vi "bangBangNavigation.vi"(0 "Game":refnum<class "Game.lvclass">, 1 "RobotRef":refnum<class "Robot.lvclass">[](array[class]), 5 "error in (no error)":errorcluster) -> (16 "RoboRef":refnum<class "Robot.lvclass">[](array[class]), 17 "NaN?":bool, 18 "NewNaN?":bool, 19 "error out":errorcluster)   [LabVIEW 2020, in "Game.lvclass"]
uses:
  Game.lvclass
  Robot_class/Robot.lvclass
  Navigation/Controls/typeOfUse.ctl
  Robot_class/Robot.lvclass/Robot.ctl
  Robot_class/Write v_ang.vi
  Robot_class/Write v_norm.vi
  Robot_class/Write v_tang.vi
  Robot_class/Read id.vi
  Robot_class/Read v_tang.vi
  Robot_class/Read v_norm.vi
  Robot_class/Read v_ang.vi
panel:
  in  "delta":dbl=0.2
  in  "desired_vtang":dbl=1.0
  in  "est_vtang":dbl=2.0
  out "array":dbl[][](array[numeric])
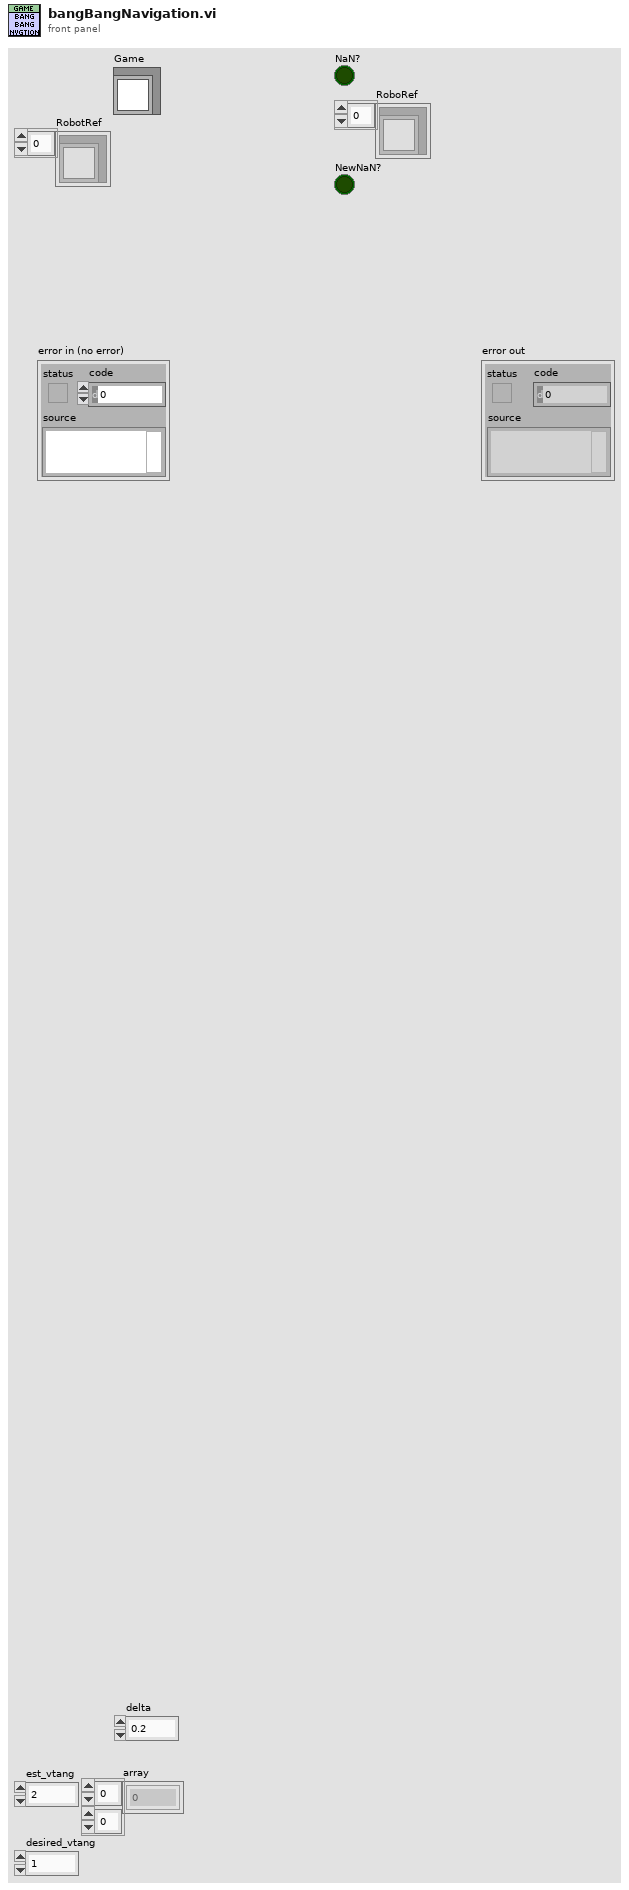
[diagram p1: front panel]
types:
  T1 = typedef "typeOfUse.ctl" = enum16{"Navigation", "grSimTest"}
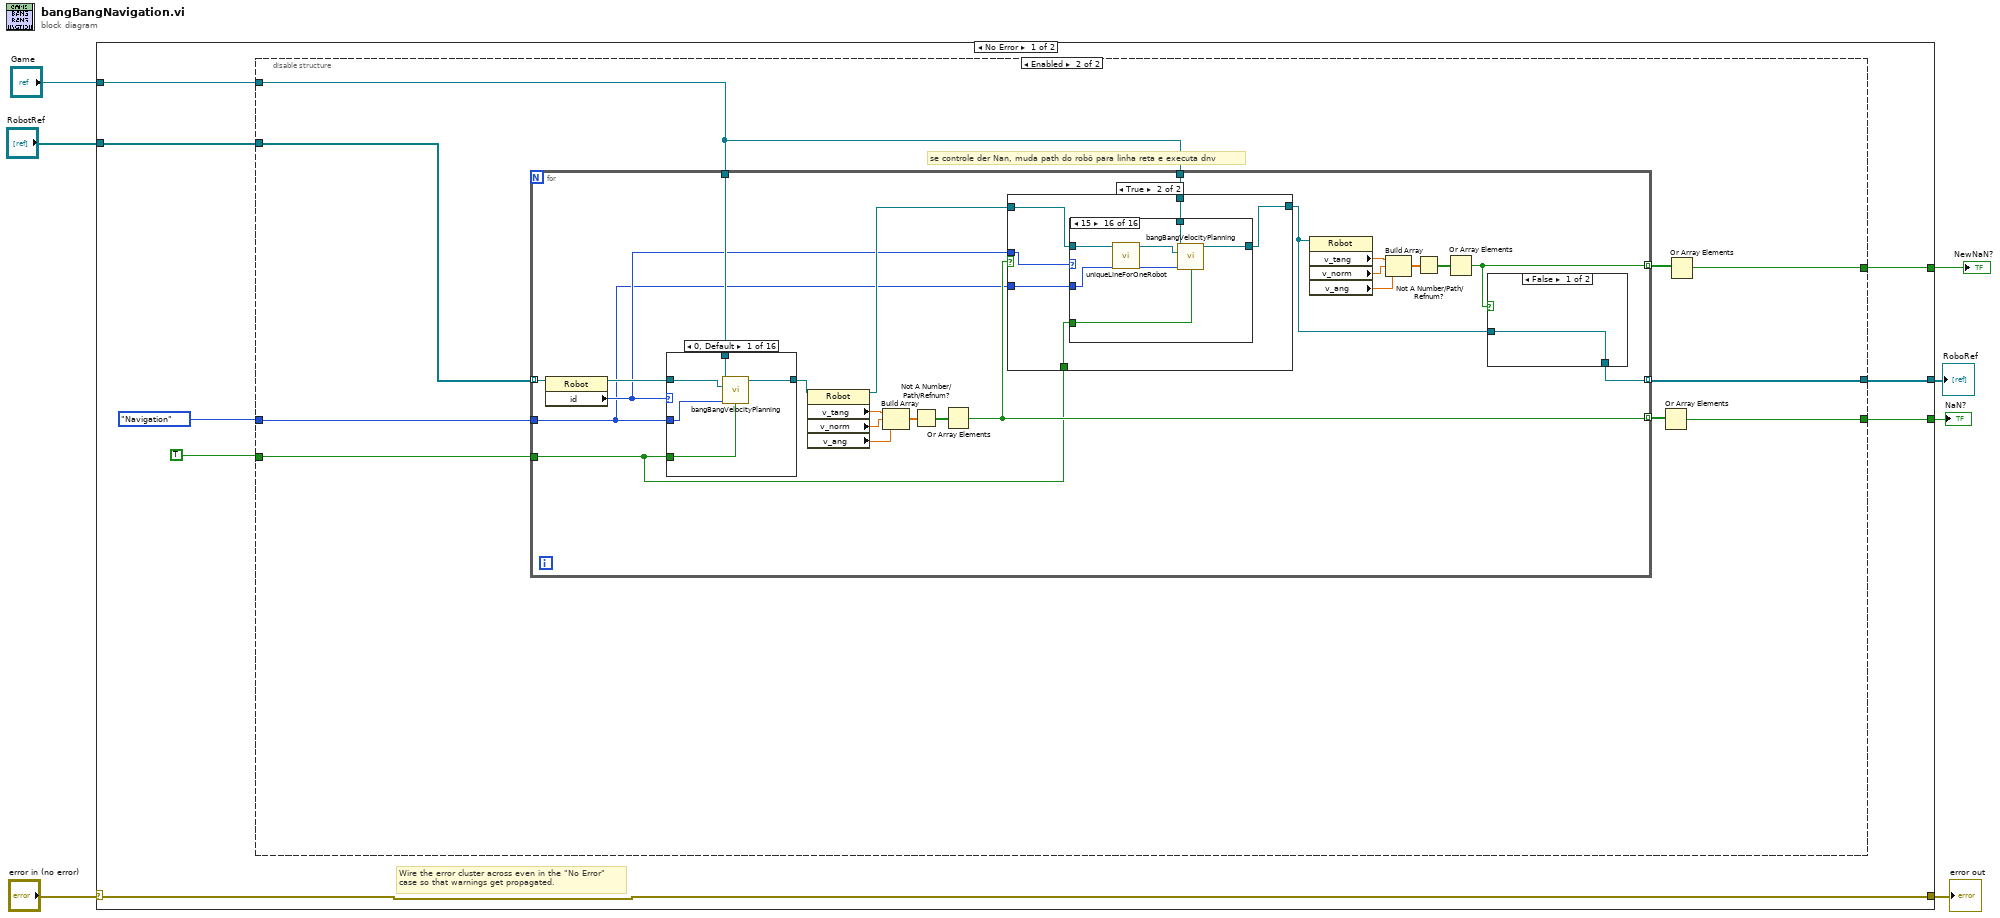
[diagram p0: block diagram]
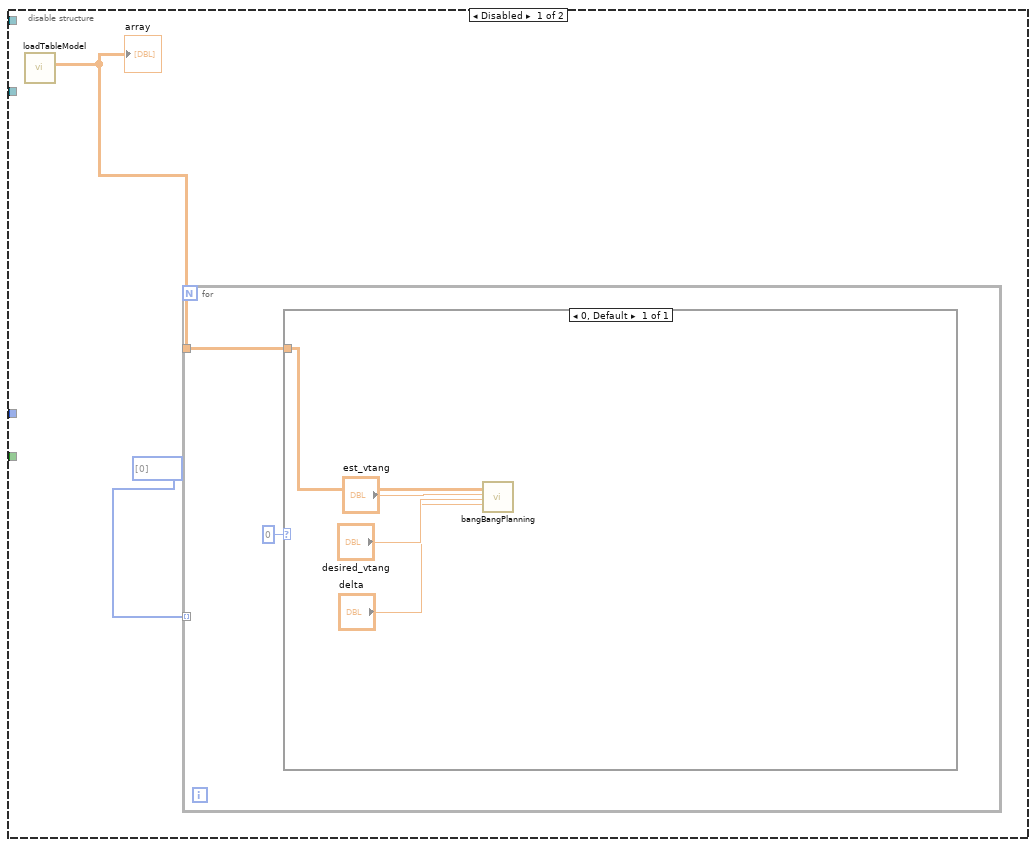
[diagram p2: hidden frame]
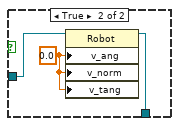
[diagram p3: hidden frame]
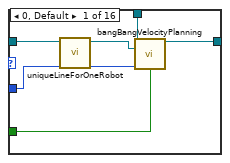
[diagram p5: hidden frame]
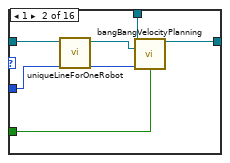
[diagram p6: hidden frame]
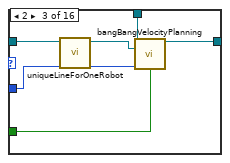
[diagram p7: hidden frame]
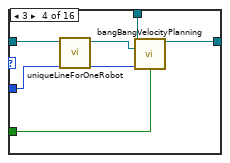
[diagram p8: hidden frame]
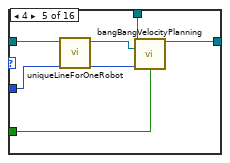
[diagram p9: hidden frame]
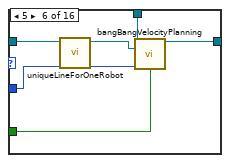
[diagram p10: hidden frame]
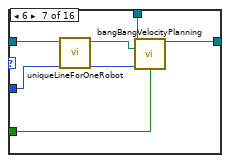
[diagram p11: hidden frame]
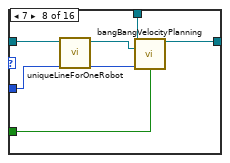
[diagram p12: hidden frame]
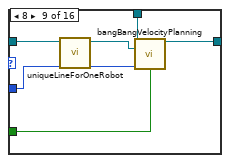
[diagram p13: hidden frame]
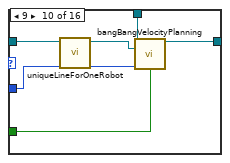
[diagram p14: hidden frame]
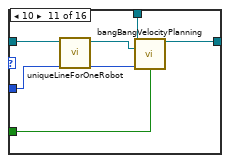
[diagram p15: hidden frame]
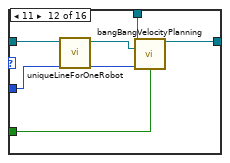
[diagram p16: hidden frame]
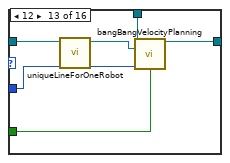
[diagram p17: hidden frame]
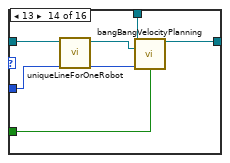
[diagram p18: hidden frame]
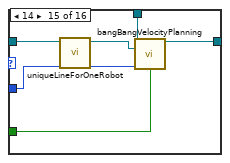
[diagram p19: hidden frame]
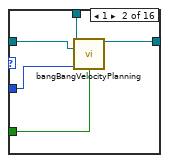
[diagram p20: hidden frame]
diagram:
  n1 = case shown="No Error" "error in (no error)" {
    selector: "error in (no error)" -> [w15 w243]
    tunnel: [w15 w243] -> w6
    tunnel: [w12 _] -> w5
    tunnel: [w11 _] -> w4
    tunnel: "RobotRef" -> [w10 _]
    tunnel: "Game" -> [w9 _]
    tunnel: [w8 _] -> w1
    frame No Error {
      # "Wire the error cluster across even in the \"No Error\"\ncase so that warnings get propagated."
      n2 = disable-structure shown="Enabled" {
        disable-tunnel: TRUE ("start") -> [_ w32]
        disable-tunnel: typeOfUse."Navigation" ("type_of_use") -> [_ w31]
        disable-tunnel: [_ w29] -> w12
        disable-tunnel: [_ w28] -> w11
        disable-tunnel: w10 -> [_ w27]
        disable-tunnel: w9 -> [_ w26]
        disable-tunnel: [_ w24] -> w8
        frame Disabled {
          n3 = call "loadTableModel.vi"() -> ("array"=w17:dbl[][])  [unwired: 9 in, 2 out]
          "array" <- w17
          n4 = for {
            tunnel: w17 -> [w19]
            tunnel: i32[] [0] -> [_] mode=indexing
            n5 = case shown="0, Default" u32 0 ("id") {
              tunnel: w19 -> [w23]
              frame 0, Default {
                n6 = call "bangBangPlanning.vi"("array"=w23, "est_vtang"="est_vtang", "desired_vtang"="desired_vtang", "delta"="delta") -> ()  [unwired: 14 in, 2 out]
              }
            }
          }
        }
        frame Enabled {
          # "se controle der Nan, muda path do robô para linha reta e executa dnv"
          n7 = for {
            tunnel: w27 -> [w55] mode=indexing
            tunnel: w32 -> [w41]
            tunnel: [w33] -> w28 mode=indexing
            tunnel: w31 -> [w42]
            tunnel: [w47] -> w30 mode=indexing
            tunnel: w26 -> [w45]
            tunnel: w26 -> [w43]
            tunnel: [w35] -> w25 mode=indexing
            n8 = property class="Robot"(reference=w55) -> (reference out=w54:refnum<class "Robot.lvclass">, "id"=w44:i32)  [unwired: 1 in, 1 out]
            n9 = case shown="0, Default" w44 {
              tunnel: w54 -> [w164 w169 w174 w179 w184 w189 w194 w199 w204 w209 w214 w219 w224 w229 w234 w239]
              tunnel: w41 -> [w167 w172 w177 w182 w187 w192 w197 w202 w207 w212 w217 w222 w227 w232 w237 w242]
              tunnel: [w166 w171 w176 w181 w186 w191 w196 w201 w206 w211 w216 w221 w226 w231 w236 w241] -> w53
              tunnel: w42 -> [w165 w170 w175 w180 w185 w190 w195 w200 w205 w210 w215 w220 w225 w230 w235 w240]
              tunnel: w45 -> [w163 w168 w173 w178 w183 w188 w193 w198 w203 w208 w213 w218 w223 w228 w233 w238]
              frame 0, Default {
                n10 = call "bangBangVelocityPlanning.vi"("Game"=w163, "Robot in"=w164, "type_of_use"=w165, "start"=w167) -> ("Robot out"=w166:refnum<class "Robot.lvclass">)  [unwired: 9 in, 2 out]
              }
              frame 1 {
                n11 = call "bangBangVelocityPlanning.vi"("Game"=w168, "Robot in"=w169, "type_of_use"=w170, "start"=w172) -> ("Robot out"=w171:refnum<class "Robot.lvclass">)  [unwired: 9 in, 2 out]
              }
              frame 2 {
                n12 = call "bangBangVelocityPlanning.vi"("Game"=w173, "Robot in"=w174, "type_of_use"=w175, "start"=w177) -> ("Robot out"=w176:refnum<class "Robot.lvclass">)  [unwired: 9 in, 2 out]
              }
              frame 3 {
                n13 = call "bangBangVelocityPlanning.vi"("Game"=w178, "Robot in"=w179, "type_of_use"=w180, "start"=w182) -> ("Robot out"=w181:refnum<class "Robot.lvclass">)  [unwired: 9 in, 2 out]
              }
              frame 4 {
                n14 = call "bangBangVelocityPlanning.vi"("Game"=w183, "Robot in"=w184, "type_of_use"=w185, "start"=w187) -> ("Robot out"=w186:refnum<class "Robot.lvclass">)  [unwired: 9 in, 2 out]
              }
              frame 5 {
                n15 = call "bangBangVelocityPlanning.vi"("Game"=w188, "Robot in"=w189, "type_of_use"=w190, "start"=w192) -> ("Robot out"=w191:refnum<class "Robot.lvclass">)  [unwired: 9 in, 2 out]
              }
              frame 6 {
                n16 = call "bangBangVelocityPlanning.vi"("Game"=w193, "Robot in"=w194, "type_of_use"=w195, "start"=w197) -> ("Robot out"=w196:refnum<class "Robot.lvclass">)  [unwired: 9 in, 2 out]
              }
              frame 7 {
                n17 = call "bangBangVelocityPlanning.vi"("Game"=w198, "Robot in"=w199, "type_of_use"=w200, "start"=w202) -> ("Robot out"=w201:refnum<class "Robot.lvclass">)  [unwired: 9 in, 2 out]
              }
              frame 8 {
                n18 = call "bangBangVelocityPlanning.vi"("Game"=w203, "Robot in"=w204, "type_of_use"=w205, "start"=w207) -> ("Robot out"=w206:refnum<class "Robot.lvclass">)  [unwired: 9 in, 2 out]
              }
              frame 9 {
                n19 = call "bangBangVelocityPlanning.vi"("Game"=w208, "Robot in"=w209, "type_of_use"=w210, "start"=w212) -> ("Robot out"=w211:refnum<class "Robot.lvclass">)  [unwired: 9 in, 2 out]
              }
              frame 10 {
                n20 = call "bangBangVelocityPlanning.vi"("Game"=w213, "Robot in"=w214, "type_of_use"=w215, "start"=w217) -> ("Robot out"=w216:refnum<class "Robot.lvclass">)  [unwired: 9 in, 2 out]
              }
              frame 11 {
                n21 = call "bangBangVelocityPlanning.vi"("Game"=w218, "Robot in"=w219, "type_of_use"=w220, "start"=w222) -> ("Robot out"=w221:refnum<class "Robot.lvclass">)  [unwired: 9 in, 2 out]
              }
              frame 12 {
                n22 = call "bangBangVelocityPlanning.vi"("Game"=w223, "Robot in"=w224, "type_of_use"=w225, "start"=w227) -> ("Robot out"=w226:refnum<class "Robot.lvclass">)  [unwired: 9 in, 2 out]
              }
              frame 13 {
                n23 = call "bangBangVelocityPlanning.vi"("Game"=w228, "Robot in"=w229, "type_of_use"=w230, "start"=w232) -> ("Robot out"=w231:refnum<class "Robot.lvclass">)  [unwired: 9 in, 2 out]
              }
              frame 14 {
                n24 = call "bangBangVelocityPlanning.vi"("Game"=w233, "Robot in"=w234, "type_of_use"=w235, "start"=w237) -> ("Robot out"=w236:refnum<class "Robot.lvclass">)  [unwired: 9 in, 2 out]
              }
              frame 15 {
                n25 = call "bangBangVelocityPlanning.vi"("Game"=w238, "Robot in"=w239, "type_of_use"=w240, "start"=w242) -> ("Robot out"=w241:refnum<class "Robot.lvclass">)  [unwired: 9 in, 2 out]
              }
            }
            n26 = property class="Robot"(reference=w53) -> (reference out=w46:refnum<class "Robot.lvclass">, "v_tang"=w52:dbl, "v_norm"=w51:dbl, "v_ang"=w49:dbl)  [unwired: 1 in, 1 out]
            n27 = Build Array(w52, w51, w49) -> (w50:dbl[])
            n28 = Not A Number/Path/Refnum?(number/path/refnum=w50) -> (NaN/Path/Refnum?=w48:bool[])
            n29 = Or Array Elements(Boolean array=w48) -> (logical OR=w47:bool)
            n30 = case shown="True" w47 {
              tunnel: w46 -> [w60 w65]
              tunnel: [w60 w61] -> w34
              tunnel: w44 -> [_ w66]
              tunnel: w43 -> [_ w64]
              tunnel: w42 -> [_ w63]
              tunnel: w41 -> [_ w62]
              frame False {
              }
              frame True {
                n31 = case shown="15" w66 {
                  tunnel: w65 -> [w68 w74 w80 w86 w92 w98 w104 w110 w116 w122 w128 w134 w140 w146 w152 w158]
                  tunnel: w62 -> [w72 w78 w84 w90 w96 w102 w108 w114 w120 w126 w132 w138 w144 w150 w156 w162]
                  tunnel: [w71 w77 w83 w89 w95 w101 w107 w113 w119 w125 w131 w137 w143 w149 w155 w161] -> w61
                  tunnel: w63 -> [w70 w76 w82 w88 w94 w100 w106 w112 w118 w124 w130 w136 w142 w148 w154 w160]
                  tunnel: w64 -> [w69 w75 w81 w87 w93 w99 w105 w111 w117 w123 w129 w135 w141 w147 w153 w159]
                  frame 0, Default {
                    n32 = call "uniqueLineForOneRobot.vi"("Robot in"=w68) -> ("Robot out"=w67:refnum<class "Robot.lvclass">)  [unwired: 10 in]
                    n33 = call "bangBangVelocityPlanning.vi"("Game"=w69, "Robot in"=w67, "type_of_use"=w70, "start"=w72) -> ("Robot out"=w71:refnum<class "Robot.lvclass">)  [unwired: 9 in, 2 out]
                  }
                  frame 1 {
                    n34 = call "uniqueLineForOneRobot.vi"("Robot in"=w74) -> ("Robot out"=w73:refnum<class "Robot.lvclass">)  [unwired: 10 in]
                    n35 = call "bangBangVelocityPlanning.vi"("Game"=w75, "Robot in"=w73, "type_of_use"=w76, "start"=w78) -> ("Robot out"=w77:refnum<class "Robot.lvclass">)  [unwired: 9 in, 2 out]
                  }
                  frame 2 {
                    n36 = call "uniqueLineForOneRobot.vi"("Robot in"=w80) -> ("Robot out"=w79:refnum<class "Robot.lvclass">)  [unwired: 10 in]
                    n37 = call "bangBangVelocityPlanning.vi"("Game"=w81, "Robot in"=w79, "type_of_use"=w82, "start"=w84) -> ("Robot out"=w83:refnum<class "Robot.lvclass">)  [unwired: 9 in, 2 out]
                  }
                  frame 3 {
                    n38 = call "uniqueLineForOneRobot.vi"("Robot in"=w86) -> ("Robot out"=w85:refnum<class "Robot.lvclass">)  [unwired: 10 in]
                    n39 = call "bangBangVelocityPlanning.vi"("Game"=w87, "Robot in"=w85, "type_of_use"=w88, "start"=w90) -> ("Robot out"=w89:refnum<class "Robot.lvclass">)  [unwired: 9 in, 2 out]
                  }
                  frame 4 {
                    n40 = call "uniqueLineForOneRobot.vi"("Robot in"=w92) -> ("Robot out"=w91:refnum<class "Robot.lvclass">)  [unwired: 10 in]
                    n41 = call "bangBangVelocityPlanning.vi"("Game"=w93, "Robot in"=w91, "type_of_use"=w94, "start"=w96) -> ("Robot out"=w95:refnum<class "Robot.lvclass">)  [unwired: 9 in, 2 out]
                  }
                  frame 5 {
                    n42 = call "uniqueLineForOneRobot.vi"("Robot in"=w98) -> ("Robot out"=w97:refnum<class "Robot.lvclass">)  [unwired: 10 in]
                    n43 = call "bangBangVelocityPlanning.vi"("Game"=w99, "Robot in"=w97, "type_of_use"=w100, "start"=w102) -> ("Robot out"=w101:refnum<class "Robot.lvclass">)  [unwired: 9 in, 2 out]
                  }
                  frame 6 {
                    n44 = call "uniqueLineForOneRobot.vi"("Robot in"=w104) -> ("Robot out"=w103:refnum<class "Robot.lvclass">)  [unwired: 10 in]
                    n45 = call "bangBangVelocityPlanning.vi"("Game"=w105, "Robot in"=w103, "type_of_use"=w106, "start"=w108) -> ("Robot out"=w107:refnum<class "Robot.lvclass">)  [unwired: 9 in, 2 out]
                  }
                  frame 7 {
                    n46 = call "uniqueLineForOneRobot.vi"("Robot in"=w110) -> ("Robot out"=w109:refnum<class "Robot.lvclass">)  [unwired: 10 in]
                    n47 = call "bangBangVelocityPlanning.vi"("Game"=w111, "Robot in"=w109, "type_of_use"=w112, "start"=w114) -> ("Robot out"=w113:refnum<class "Robot.lvclass">)  [unwired: 9 in, 2 out]
                  }
                  frame 8 {
                    n48 = call "uniqueLineForOneRobot.vi"("Robot in"=w116) -> ("Robot out"=w115:refnum<class "Robot.lvclass">)  [unwired: 10 in]
                    n49 = call "bangBangVelocityPlanning.vi"("Game"=w117, "Robot in"=w115, "type_of_use"=w118, "start"=w120) -> ("Robot out"=w119:refnum<class "Robot.lvclass">)  [unwired: 9 in, 2 out]
                  }
                  frame 9 {
                    n50 = call "uniqueLineForOneRobot.vi"("Robot in"=w122) -> ("Robot out"=w121:refnum<class "Robot.lvclass">)  [unwired: 10 in]
                    n51 = call "bangBangVelocityPlanning.vi"("Game"=w123, "Robot in"=w121, "type_of_use"=w124, "start"=w126) -> ("Robot out"=w125:refnum<class "Robot.lvclass">)  [unwired: 9 in, 2 out]
                  }
                  frame 10 {
                    n52 = call "uniqueLineForOneRobot.vi"("Robot in"=w128) -> ("Robot out"=w127:refnum<class "Robot.lvclass">)  [unwired: 10 in]
                    n53 = call "bangBangVelocityPlanning.vi"("Game"=w129, "Robot in"=w127, "type_of_use"=w130, "start"=w132) -> ("Robot out"=w131:refnum<class "Robot.lvclass">)  [unwired: 9 in, 2 out]
                  }
                  frame 11 {
                    n54 = call "uniqueLineForOneRobot.vi"("Robot in"=w134) -> ("Robot out"=w133:refnum<class "Robot.lvclass">)  [unwired: 10 in]
                    n55 = call "bangBangVelocityPlanning.vi"("Game"=w135, "Robot in"=w133, "type_of_use"=w136, "start"=w138) -> ("Robot out"=w137:refnum<class "Robot.lvclass">)  [unwired: 9 in, 2 out]
                  }
                  frame 12 {
                    n56 = call "uniqueLineForOneRobot.vi"("Robot in"=w140) -> ("Robot out"=w139:refnum<class "Robot.lvclass">)  [unwired: 10 in]
                    n57 = call "bangBangVelocityPlanning.vi"("Game"=w141, "Robot in"=w139, "type_of_use"=w142, "start"=w144) -> ("Robot out"=w143:refnum<class "Robot.lvclass">)  [unwired: 9 in, 2 out]
                  }
                  frame 13 {
                    n58 = call "uniqueLineForOneRobot.vi"("Robot in"=w146) -> ("Robot out"=w145:refnum<class "Robot.lvclass">)  [unwired: 10 in]
                    n59 = call "bangBangVelocityPlanning.vi"("Game"=w147, "Robot in"=w145, "type_of_use"=w148, "start"=w150) -> ("Robot out"=w149:refnum<class "Robot.lvclass">)  [unwired: 9 in, 2 out]
                  }
                  frame 14 {
                    n60 = call "uniqueLineForOneRobot.vi"("Robot in"=w152) -> ("Robot out"=w151:refnum<class "Robot.lvclass">)  [unwired: 10 in]
                    n61 = call "bangBangVelocityPlanning.vi"("Game"=w153, "Robot in"=w151, "type_of_use"=w154, "start"=w156) -> ("Robot out"=w155:refnum<class "Robot.lvclass">)  [unwired: 9 in, 2 out]
                  }
                  frame 15 {
                    n62 = call "uniqueLineForOneRobot.vi"("Robot in"=w158) -> ("Robot out"=w157:refnum<class "Robot.lvclass">)  [unwired: 10 in]
                    n63 = call "bangBangVelocityPlanning.vi"("Game"=w159, "Robot in"=w157, "type_of_use"=w160, "start"=w162) -> ("Robot out"=w161:refnum<class "Robot.lvclass">)  [unwired: 9 in, 2 out]
                  }
                }
              }
            }
            n64 = property class="Robot"(reference=w34) -> ("v_tang"=w40:dbl, "v_norm"=w39:dbl, "v_ang"=w37:dbl)  [unwired: 1 in, 2 out]
            n65 = Build Array(w40, w39, w37) -> (w38:dbl[])
            n66 = Not A Number/Path/Refnum?(number/path/refnum=w38) -> (NaN/Path/Refnum?=w36:bool[])
            n67 = Or Array Elements(Boolean array=w36) -> (logical OR=w35:bool)
            n68 = case shown="False" w35 {
              tunnel: w34 -> [w56 w59]
              tunnel: [w56 w57] -> w33
              frame False {
              }
              frame True {
                w58 = 0.0 ("v_ang")
                n69 = property class="Robot"(reference=w59, "v_ang"=w58, "v_norm"=w58, "v_tang"=w58) -> (reference out=w57:refnum<class "Robot.lvclass">)  [unwired: 1 in, 1 out]
              }
            }
          }
          n70 = Or Array Elements(Boolean array=w30) -> (logical OR=w29:bool)
          n71 = Or Array Elements(Boolean array=w25) -> (logical OR=w24:bool)
        }
      }
    }
    frame Error {
    }
  }
  "error out" <- w6
  "NaN?" <- w5
  "RoboRef" <- w4
  "NewNaN?" <- w1
